vi "Save Output2.vi"(7 "Reset":bool=TRUE, 8 "input valid":bool=TRUE, 11 "Data in":fxp<+/-,32,14>[](array[numeric])=[0.0, 0.0]) -> ()   [LabVIEW 2018]
uses:
  <vilib>/rvi/Emulation/niFpgaSctlEmulationGetInTimedLoop.vi
  <vilib>/rvi/Memory/Memory_Emulation/nirvimemoryFastEmulation.vi
  <vilib>/rvi/Memory/Memory_Emulation/nirvimemoryEmulation.vi
  <vilib>/rvi/Emulation/niFpgaEmulationIsFPGAContextNoSignature.vi
  <vilib>/rvi/DataTransferAndStorage/Container/Common/niFpgaContainerGetUniqueNameForEmu.vi
  <vilib>/rvi/Emulation/niFpgaProcessEmulError.vi
  <vilib>/rvi/errors/nirviReportUnexpectedCaseInternalError (U32).vi
  <vilib>/rvi/DataTransferAndStorage/Container/XNode/niFpgaContainer.xnode
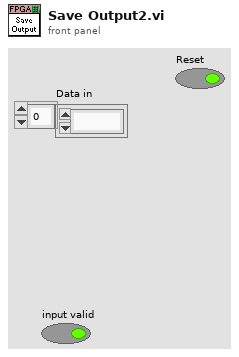
[diagram p1: front panel]
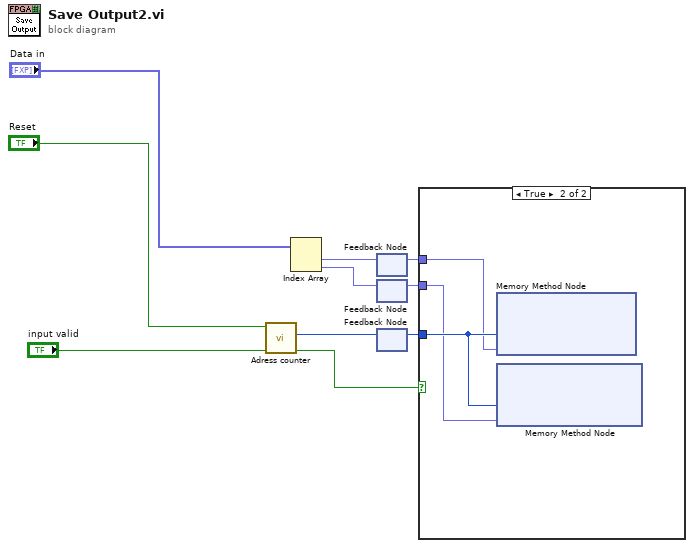
[diagram p0: block diagram]
diagram:
  n1 = call "Adress counter.vi"("input valid"="input valid", "Reset"="Reset") -> ("output valid"=w1:bool, "Address"=w8:u32)  [unwired: 8 in]
  n2 = Index Array(array="Data in") -> (element #1=w4:fxp<+/-,32,14>, element #2=w5:fxp<+/-,32,14>)  [unwired: 2 in]
  n3 = feedback #1() -> (w2:fxp<+/-,32,14>)  [unwired: 1 in]
  n4 = feedback-in #1(w4) -> ()
  n5 = feedback #2() -> (w3:fxp<+/-,32,14>)  [unwired: 1 in]
  n6 = feedback-in #2(w5) -> ()
  n7 = feedback #3() -> (w7:u32)  [unwired: 1 in]
  n8 = feedback-in #3(w8) -> ()
  n9 = case shown="True" w1 {
    tunnel: w7 -> [_ w13]
    tunnel: w3 -> [_ w12]
    tunnel: w2 -> [_ w11]
    frame False {
    }
    frame True {
      n10 = xnode ("Memory Method Node")("Address"=w13, "Data"=w11) -> ()  [unwired: 1 in, 1 out]
      n11 = xnode ("Memory Method Node")("Address"=w13, "Data"=w12) -> ()  [unwired: 1 in, 1 out]
    }
  }
